vi "数据查询_仪器数据.vi"() -> ()   [LabVIEW 2016]
uses:
  <vilib>/Utility/miscctls.llb/LVRowAndColumnUnsignedTypeDef.ctl
  <vilib>/Utility/miscctls.llb/LVPointTypeDef.ctl
  <userlib>/_OpenG.lib/array/array.llb/Sort 2D Array (String)__ogtk.vi
panel:
  out "布尔":bool
  in  "页":i32 format="第%.0f页"
  in  "每页条数":i32=20
  in  "向后按钮":bool
  in  "向前按钮":bool
  in  "下拉列表":string(xcontrol)
  in  "导出":bool
  out "分钟小时":string(combo)="实时数据"
  out "工作类型":string(combo)="全部数据"
  in  "查询":bool
  in  "结束日期":string="2050/01/01"
  in  "起始日期":string="2010/01/01"
  out "数据表":string[][](table)
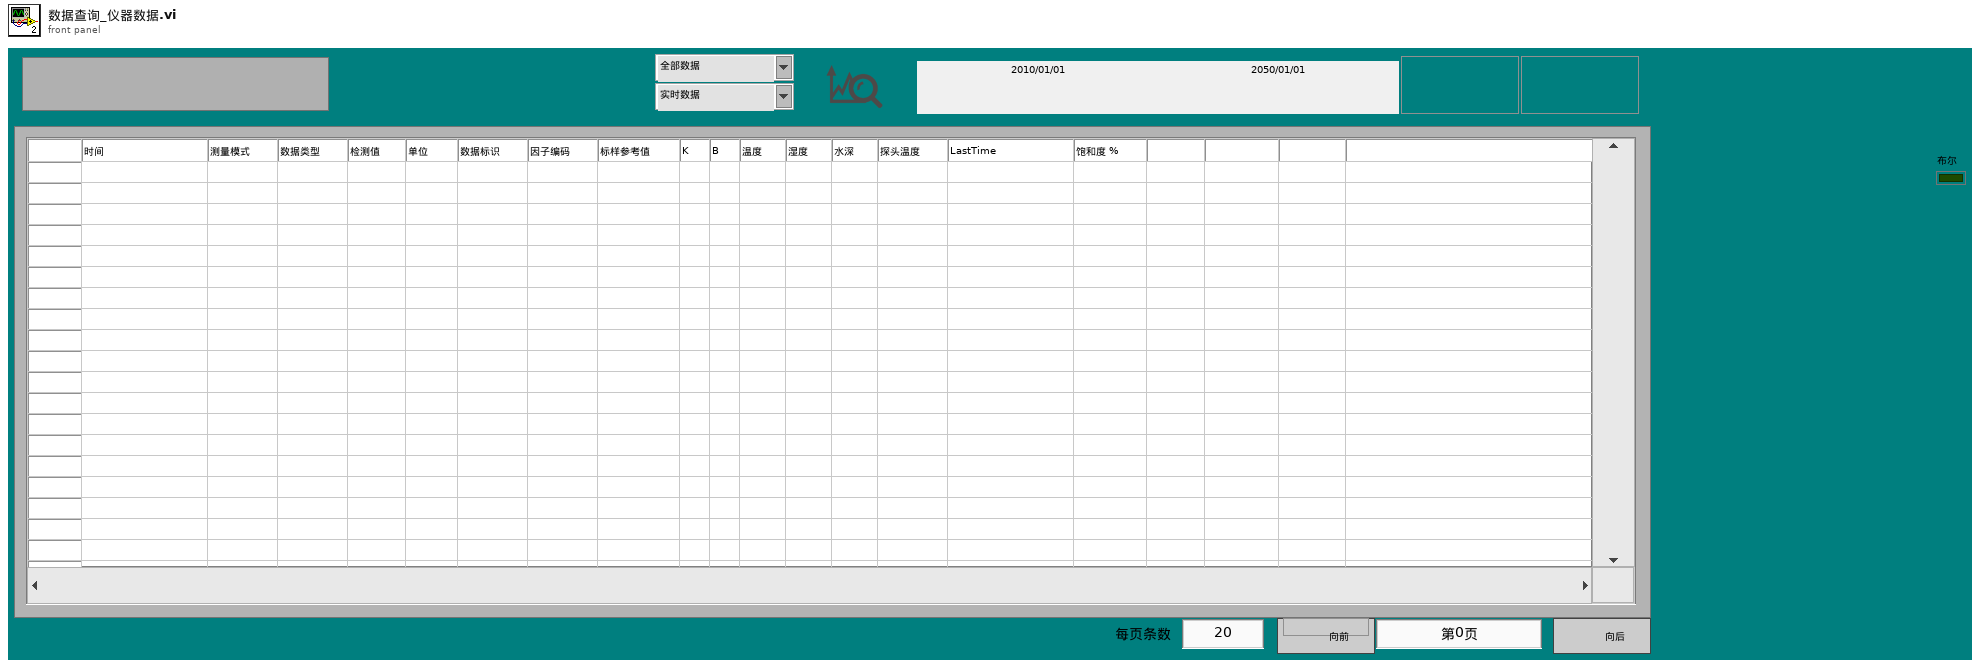
[diagram p1: front panel]
types:
  T1 = enum8{"Enabled", "Disabled", "Disabled and Grayed Out"}
  T2 = typedef "LVRowAndColumnUnsignedTypeDef.ctl" = cluster{"Row":u32, "Column":u32}
  T3 = typedef "LVPointTypeDef.ctl" = cluster{"Horizontal":i16, "Vertical":i16}
  T4 = typedef "LVDateTimeRec.ctl" = cluster{"秒数的小数部分":dbl, "秒":i32, "分":i32, "时":i32, "日":i32, "月":i32, "年":i32, "天数（周）":i32, "天数（年）":i32, "DST":i32}
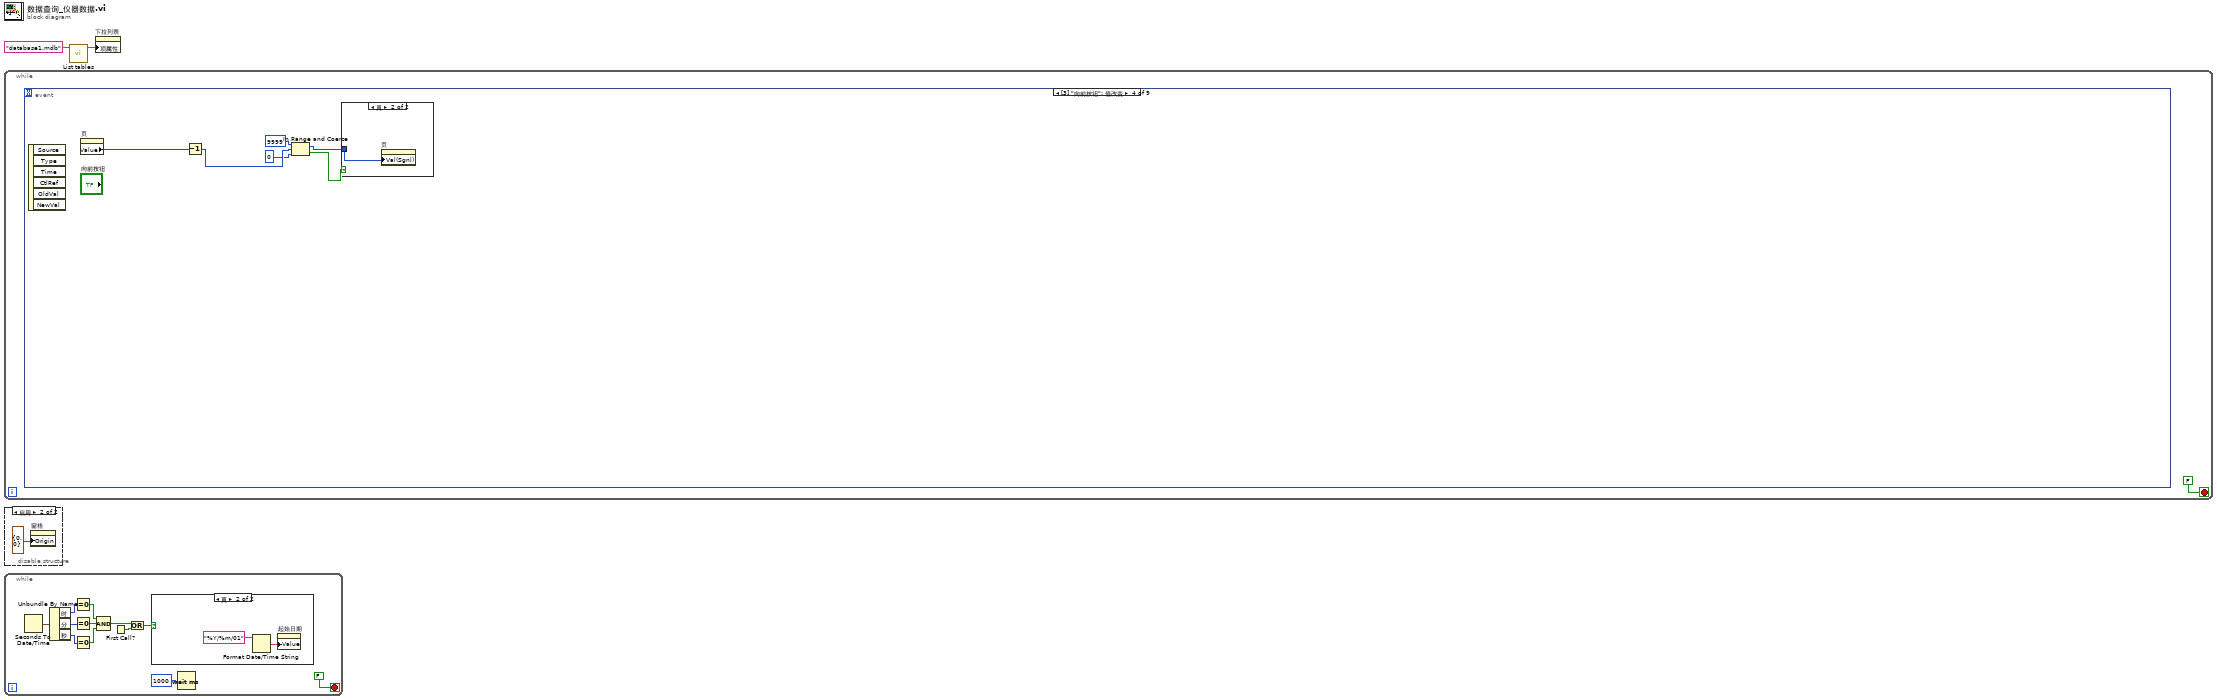
[diagram p0: block diagram]
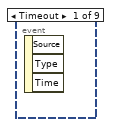
[diagram p3: hidden frame]
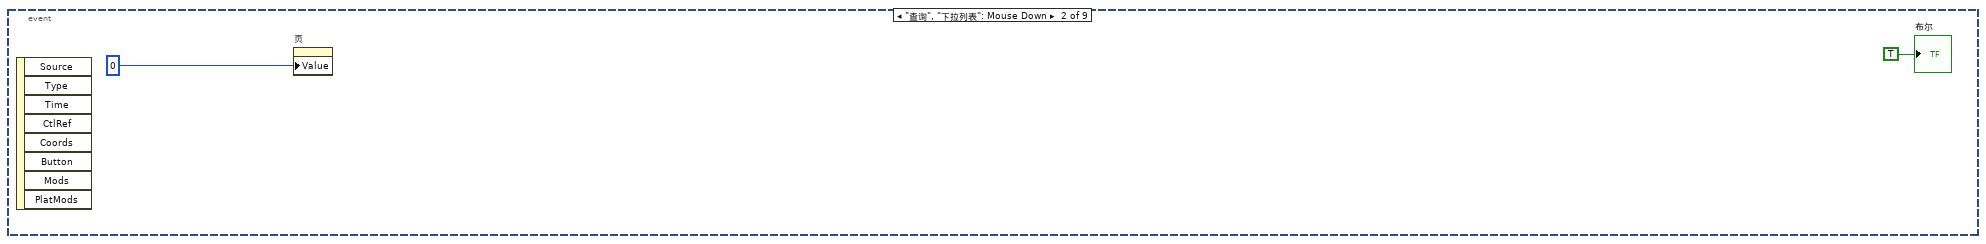
[diagram p4: hidden frame]
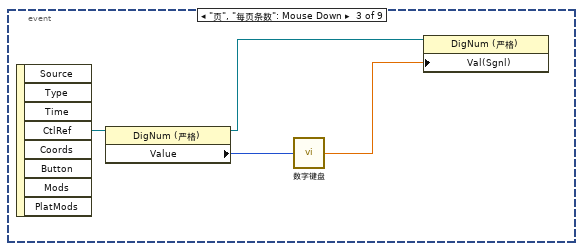
[diagram p5: hidden frame]
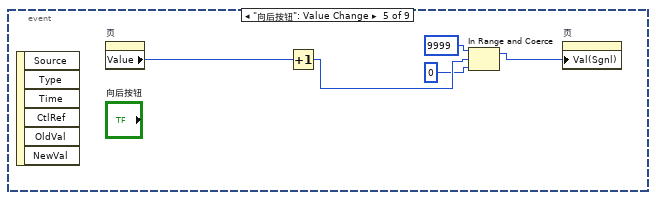
[diagram p7: hidden frame]
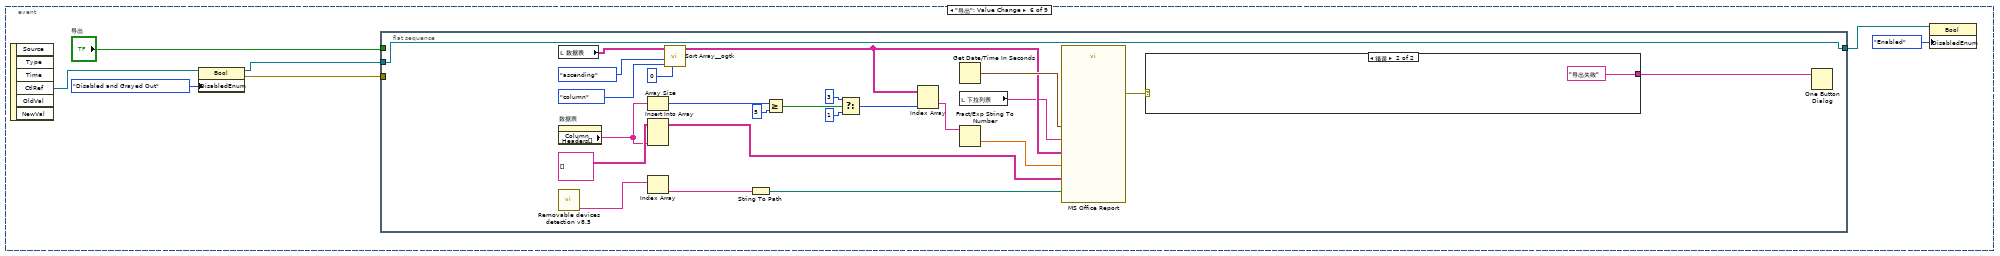
[diagram p8: hidden frame]
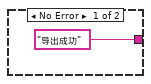
[diagram p9: hidden frame]
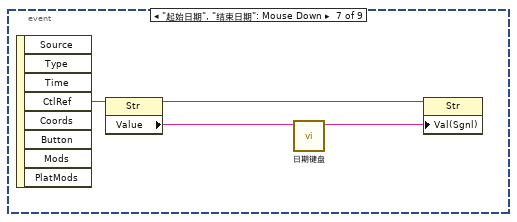
[diagram p10: hidden frame]
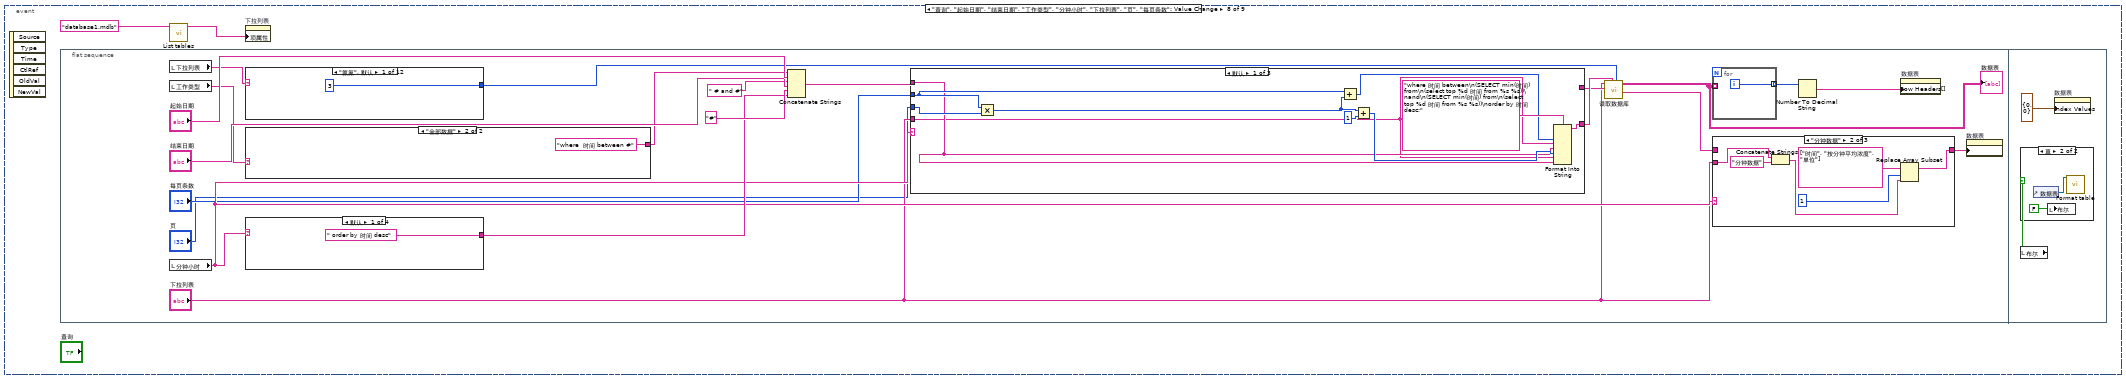
[diagram p11: hidden frame]
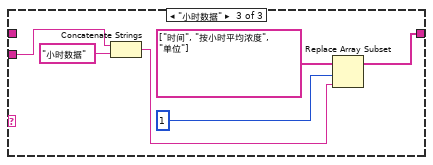
[diagram p13: hidden frame]
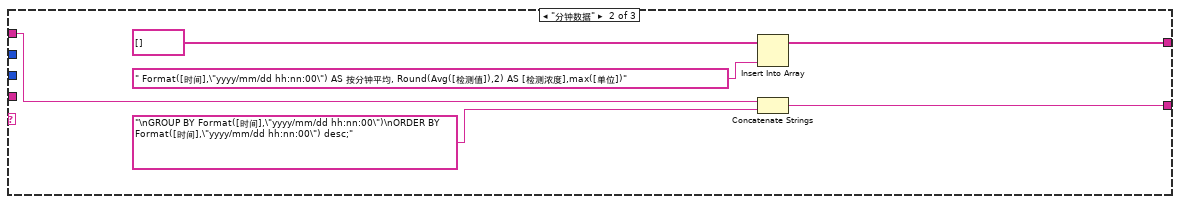
[diagram p17: hidden frame]
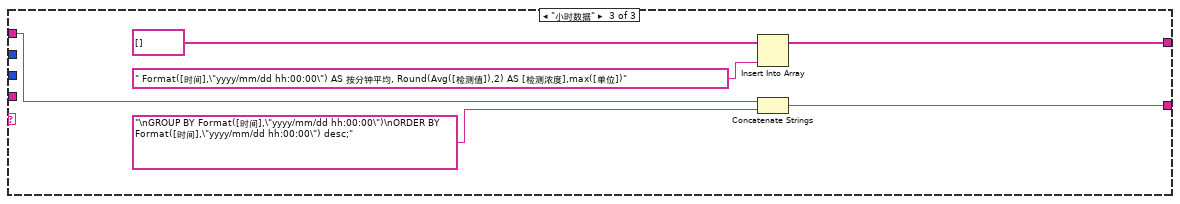
[diagram p18: hidden frame]
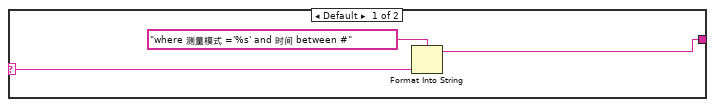
[diagram p19: hidden frame]
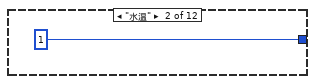
[diagram p20: hidden frame]
diagram:
  n1 = while {
    stop <- FALSE stop-if-true
    n2 = event shown="[3] \"向前按钮\": 值改变" {
      selector: _ -> [_ _ _ _ _ _ _ _ _]
      dyn-events: _ -> [_ _ _ _ _ _ _ _ _]
      timeout: _ -> [_ _ _ _ _ _ _ _ _]
      event Timeout {
        n3 = event-data() -> ()  [unwired: 1 in, 3 out]
      }
      event "查询", "下拉列表": Mouse Down {
        n4 = event-data() -> ()  [unwired: 1 in, 8 out]
        n5 = property on="页" class="DigNum (严格)"("Value"=0 ("页")) -> ()  [unwired: 2 in, 2 out]
        "布尔" <- TRUE ("布尔")
      }
      event "页", "每页条数": Mouse Down {
        n6 = event-data() -> ("CtlRef"=w6:refnum<vi>)  [unwired: 1 in, 7 out]
        n7 = property class="DigNum (严格)"(reference=w6) -> (reference out=w7:refnum<vi>, "Value"=w9:i32)  [unwired: 1 in, 1 out]
        n8 = call "数字键盘.vi"("OldNumber"=w9) -> ("NewNumber"=w8:sgl)
        n9 = property class="DigNum (严格)"(reference=w7, "Val(Sgnl)"=w8) -> ()  [unwired: 1 in, 2 out]
      }
      event "向前按钮": Value Change {
        n10 = event-data() -> ()  [unwired: 1 in, 6 out]
        n11 = property on="页" class="DigNum (严格)"() -> ("Value"=w15:i32)  [unwired: 2 in, 2 out]
        n12 = Decrement(x=w15) -> (x-1=w14:i32)
        n13 = In Range and Coerce(upper limit=9999 ("上限"), x=w14, lower limit=0 ("下限")) -> (coerced(x)=w11:i32, In Range?=w10:bool)
        n14 = case shown="真" w10 {
          tunnel: w11 -> [_ w16]
          frame False {
          }
          frame True {
            n15 = property on="页" class="DigNum (严格)"("Val(Sgnl)"=w16) -> ()  [unwired: 2 in, 2 out]
          }
        }
      }
      event "向后按钮": Value Change {
        n16 = event-data() -> ()  [unwired: 1 in, 6 out]
        n17 = property on="页" class="DigNum (严格)"() -> ("Value"=w21:i32)  [unwired: 2 in, 2 out]
        n18 = Increment(x=w21) -> (x+1=w20:i32)
        n19 = In Range and Coerce(upper limit=u32 9999 ("上限"), x=w20, lower limit=u32 0 ("下限")) -> (coerced(x)=w17:u32)  [unwired: 1 out]
        n20 = property on="页" class="DigNum (严格)"("Val(Sgnl)"=w17) -> ()  [unwired: 2 in, 2 out]
      }
      event "导出": Value Change {
        n21 = event-data() -> ("CtlRef"=w22:refnum<vi>)  [unwired: 1 in, 5 out]
        n22 = property class="Bool"(reference=w22, "DisabledEnum"=T1."Disabled and Grayed Out" ("禁用")) -> (reference out=w26:refnum<vi>, error out=w27:errorcluster)  [unwired: 1 in]
        n23 = flat-sequence {
          tunnel: w27 -> [_]
          tunnel: [w43] -> w25
          tunnel: w26 -> [w43]
          tunnel: "导出" -> [_]
          frame #0 {
            n24 = local read "数据表"() -> (w51:string[][])
            n25 = property on="数据表" class="Tbl (严格)"() -> ("Column Headers[]"=w30:string[])  [unwired: 2 in, 2 out]
            n26 = call "Removable devices detection v8.5.vi"() -> ("Removable"=w40:string[])  [unwired: 4 out]
            n27 = Array Size(array=w30) -> (size(s)=w37:i32)
            n28 = Insert Into Array(array=string[][] [], new element=w30) -> (w29:string[][])  [unwired: 2 in]
            n29 = Index Array(array=w40) -> (element=w39:string)  [unwired: 1 in]
            n30 = call-poly <userlib>:"Sort Array__ogtk.vi"("Column/Row to Sort By"=u32 0, "Sort By in"=enum16{"row", "column"}."column", "Order"=enum16{"ascending", "descending"}."ascending", "Array in"=w51) -> ("Sorted Array out"=w50:string[][])  [unwired: 4 in, 3 out]
            n31 = String To Path(string=w39) -> (path=w38:path)
            n32 = Greater Or Equal?(x=w37, y=5) -> (x >= y?=w35:bool)
            n33 = Select(t=3 ("禁用的索引 (列)"), s=w35, f=1) -> (s? t:f=w33:i32)
            n34 = Index Array(array=w50, index (col)=w33) -> (element=w46:string[])  [unwired: 1 in]
            n35 = Get Date/Time In Seconds() -> (seconds since 1Jan1904=w52:timestamp)
            n36 = local read "下拉列表"() -> (w44:string)
            n37 = Fract/Exp String To Number(string=w46) -> (number=w45:dbl[])  [unwired: 3 in, 1 out]
            n38 = call "MS Office Report"("Path to Save Report"=w38, "导出日期"=w52, "监测参数"=w44, "数据输入"=w50, "图表输入"=w45, "字段定义"=w29) -> ("error out"=w42:errorcluster)  [unwired: 20 in, 1 out]
            n39 = case shown="错误" w42 {
              tunnel: ["导出成功" ("消息") "导出失败" ("消息")] -> w41
              frame No Error {
              }
              frame Error {
              }
            }
            n40 = One Button Dialog(message=w41) -> ()  [unwired: 1 in, 1 out]
          }
        }
        n41 = property class="Bool"(reference=w25, "DisabledEnum"=T1."Enabled" ("禁用")) -> ()  [unwired: 1 in, 2 out]
      }
      event "起始日期", "结束日期": Mouse Down {
        n42 = event-data() -> ("CtlRef"=w58:refnum<vi>)  [unwired: 1 in, 7 out]
        n43 = property class="Str"(reference=w58) -> (reference out=w56:refnum<vi>, "Value"=w57:string)  [unwired: 1 in, 1 out]
        n44 = call "日期键盘.vi"("原值"=w57) -> ("x+y"=w55:string)  [unwired: 10 in]
        n45 = property class="Str"(reference=w56, "Val(Sgnl)"=w55) -> ()  [unwired: 1 in, 2 out]
      }
      event "查询", "起始日期", "结束日期", "工作类型", "分钟小时", "下拉列表", "页", "每页条数": Value Change {
        n46 = event-data() -> ()  [unwired: 1 in, 6 out]
        n47 = flat-sequence {
          frame #0 {
            n48 = local read "下拉列表"() -> (w74:string)
            n49 = local read "工作类型"() -> (w72:string)
            n50 = local read "分钟小时"() -> (w66:string)
            n51 = case shown="\"氨氮\", 默认" w74 {
              tunnel: [i16 3 ("精度(6)") i16 1 ("精度(6)") i16 2 ("精度(6)") i16 2 ("精度(6)") i16 2 ("精度(6)") i16 2 ("精度(6)") i16 2 ("精度(6)") i16 2 ("精度(6)") i16 3 ("精度(6)") i16 2 ("精度(6)") i16 2 ("精度(6)") i16 2 ("精度(6)")] -> w73
              frame "氨氮", Default {
              }
              frame "水温" {
              }
              frame "pH" {
              }
              frame "溶解氧" {
              }
              frame "电导率" {
              }
              frame "浊度" {
              }
              frame "藻密度" {
              }
              frame "叶绿素a" {
              }
              frame "总磷" {
              }
              frame "总氮" {
              }
              frame "CodCr" {
              }
              frame "CodMn" {
              }
            }
            n52 = case shown="\"全部数据\"" w72 {
              selector: w72 -> [w120 _]
              tunnel: [w118 "where  时间 between #" ("condition")] -> w71
              frame Default {
                n53 = Format Into String(format string="where 测量模式 ='%s' and 时间 between #" ("condition"), w120) -> (resulting string=w118:string)  [unwired: 2 in, 1 out]
              }
              frame "全部数据" {
              }
            }
            n54 = case shown="默认" w66 {
              tunnel: [" order by 时间 desc" ("字符串") _ _ _] -> w70
              frame Default {
              }
              frame "分钟数据" {
              }
              frame "小时数据" {
              }
              frame "真" {
              }
            }
            n55 = Concatenate Strings(w71, "起始日期", " # and #" ("condition"), "结束日期", "#" ("condition"), w70) -> (w69:string)
            n56 = case shown="默认" w66 {
              tunnel: [_ w110 w112] -> w67
              tunnel: w69 -> [w97 w108 w114]
              tunnel: [w100 w107 w113] -> w68
              tunnel: "下拉列表" -> [w96 _ _]
              tunnel: "每页条数" -> [w99 _ _]
              tunnel: "页" -> [w98 _ _]
              frame Default {
                n57 = Multiply(x=w99, y=w98) -> (x*y=w104:i32)
                n58 = Add(x=w99, y=w104) -> (x+y=w102:i32)
                n59 = Add(x=w104, y=u32 1) -> (x+y=w101:u32)
                n60 = Format Into String(format string="where 时间 between\n(SELECT min(时间) from\n(select top %d 时间 from %s %s))\nand\n(SELECT min(时间) from\n(select top %d 时间 from %s %s))\norder by 时间 desc;" ("格式字符串"), w102, w96, w97, w101, w96, w97) -> (resulting string=w100:string)  [unwired: 2 in, 1 out]
              }
              frame "分钟数据" {
                n61 = Insert Into Array(array=string[] [] ("显示项"), new element=" Format([时间],\"yyyy/mm/dd hh:nn:00\") AS 按分钟平均, Round(Avg([检测值]),2) AS [检测浓度],max([单位])" ("新元素/子数组")) -> (w110:string[])  [unwired: 1 in]
                n62 = Concatenate Strings(w108, "\nGROUP BY Format([时间],\"yyyy/mm/dd hh:nn:00\")\nORDER BY Format([时间],\"yyyy/mm/dd hh:nn:00\") desc;" ("字符串")) -> (w107:string)
              }
              frame "小时数据" {
                n63 = Insert Into Array(array=string[] [] ("显示项"), new element=" Format([时间],\"yyyy/mm/dd hh:00:00\") AS 按分钟平均, Round(Avg([检测值]),2) AS [检测浓度],max([单位])" ("新元素/子数组")) -> (w112:string[])  [unwired: 1 in]
                n64 = Concatenate Strings(w114, "\nGROUP BY Format([时间],\"yyyy/mm/dd hh:00:00\")\nORDER BY Format([时间],\"yyyy/mm/dd hh:00:00\") desc;" ("字符串")) -> (w113:string)
              }
            }
            n65 = call "读取数据库.vi"("精度(6)"=w73, "condition"=w68, "显示项"=w67, "组合框"="下拉列表") -> ("columns"=w65:string[], "表格"=w77:string[][])  [unwired: 4 in, 2 out]
            "数据表" <- w77
            n66 = for {
              tunnel: w77 -> [_] mode=indexing
              tunnel: [w134] -> w76 mode=indexing
              i -> [w134]
            }
            n67 = case shown="\"分钟数据\"" w66 {
              tunnel: w65 -> [w82 _ _]
              tunnel: [w82 w86 w90] -> w64
              tunnel: "下拉列表" -> [_ w85 w91]
              frame Default {
              }
              frame "分钟数据" {
                n68 = Concatenate Strings(w85, "分钟数据" ("字符串")) -> (w83:string)
                n69 = Replace Array Subset(array=string[] ["时间", "按分钟平均浓度", "单位"] ("columns"), new element=w83, index=1 ("索引")) -> (w86:string[])
              }
              frame "小时数据" {
                n70 = Concatenate Strings(w91, "小时数据" ("字符串")) -> (w92:string)
                n71 = Replace Array Subset(array=string[] ["时间", "按小时平均浓度", "单位"] ("columns"), new element=w92, index=1 ("索引")) -> (w90:string[])
              }
            }
            n72 = Number To Decimal String(number=w76) -> (decimal integer string=w75:string[])  [unwired: 1 in]
            n73 = property on="数据表" class="Tbl (严格)"("Row Headers[]"=w75) -> ()  [unwired: 2 in, 2 out]
            n74 = property on="数据表" class="Tbl (严格)"("Column Headers[]"=w64) -> ()  [unwired: 2 in, 2 out]
          }
          frame #1 {
            n75 = local read "布尔"() -> (w135:bool)
            n76 = case shown="真" w135 {
              frame False {
              }
              frame True {
                n77 = control-ref of="数据表"() -> (w138:refnum<vi>)
                n78 = local write "布尔"(FALSE ("布尔")) -> ()
                n79 = call "Format table.vi"("Table输入"=w138) -> ()  [unwired: 11 in]
              }
            }
            n80 = property on="数据表" class="Tbl (严格)"("Index Values"=T2 {"Row"=0, "Column"=0} ("索引值")) -> ()  [unwired: 2 in, 2 out]
          }
        }
        n81 = call "List tables.vi"("database"="database1.mdb") -> ("tables"=w59:string[])  [unwired: 9 in, 1 out]
        n82 = property on="下拉列表" class="下拉列表 (严格)"("项属性"=w59) -> ()  [unwired: 2 in, 2 out]
      }
      event "工作类型", "分钟小时": Mouse Down {
        n83 = event-data() -> ()  [unwired: 1 in, 8 out]
        n84 = call "数据查询筛选.vi"() -> ("分钟小时"=→"分钟小时":string, "工作类型"=→"工作类型":string)  [unwired: 10 in]
      }
    }
  }
  n85 = disable-structure shown="启用" {
    frame Disabled {
    }
    frame Enabled {
      n86 = property on="窗格" class="Pane"("Origin"=T3 {"Horizontal"=0, "Vertical"=0} ("原点")) -> ()  [unwired: 2 in, 2 out]
    }
  }
  n87 = while {
    stop <- FALSE stop-if-true
    n88 = Seconds To Date/Time() -> (date time rec=w153:T4)  [unwired: 2 in]
    n89 = Unbundle By Name(w153) -> ("时"=w152:i32, "分"=w151:i32, "秒"=w150:i32)
    n90 = Equal To 0?(x=w152) -> (x = 0?=w149:bool)
    n91 = Equal To 0?(x=w151) -> (x = 0?=w148:bool)
    n92 = Equal To 0?(x=w150) -> (x = 0?=w147:bool)
    n93 = Compound Arithmetic op=AND ("复合运算")(w149, w148, w147) -> (w144:bool)
    n94 = First Call?() -> (First Call?: T/F=w142:bool)
    n95 = Or(x=w144, y=w142) -> (x .or. y?=w143:bool)
    n96 = case shown="真" w143 {
      frame False {
      }
      frame True {
        n97 = Format Date/Time String(time format string (%c)="%Y/%m/01" ("时间格式字符串(%c)")) -> (date/time string=w154:string)  [unwired: 2 in]
        n98 = property on="起始日期" class="Str"("Value"=w154) -> ()  [unwired: 2 in, 2 out]
      }
    }
    n99 = Wait (ms)(milliseconds to wait=u32 1000 ("等待时间（毫秒）")) -> ()  [unwired: 1 out]
  }
  n100 = call "List tables.vi"("database"="database1.mdb") -> ("tables"=w1:string[])  [unwired: 9 in, 1 out]
  n101 = property on="下拉列表" class="下拉列表 (严格)"("项属性"=w1) -> ()  [unwired: 2 in, 2 out]
